vi "Write configuration.vi"(8 "error in":errorcluster, 10 "configuration":refnum<class "NISE_CEF_serializable configuration.lvclass">, 11 "cfg cRIO root in":refnum<class "cfg cRIO root.lvclass">) -> (0 "error out":errorcluster, 3 "cfg cRIO root out":refnum<class "cfg cRIO root.lvclass">)   [LabVIEW 2013, in "cfg cRIO root.lvclass"]
uses:
  cfg cRIO root.lvclass
  criocfg/crio configuration.lvclass
  CEF_TreeControl/serializable configuration/NISE_CEF_serializable configuration.lvclass
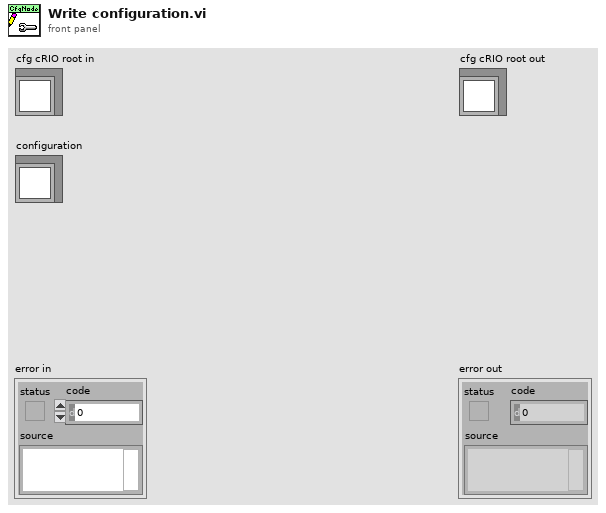
[diagram p1: front panel]
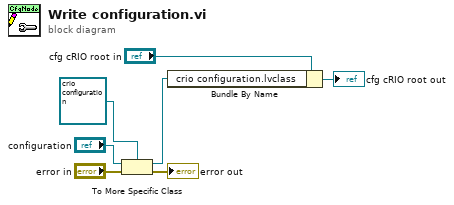
[diagram p0: block diagram]
diagram:
  n1 = To More Specific Class(target class=refnum<class "crio configuration.lvclass"> refnum ("crio configuration.lvclass"), reference="configuration", error in="error in") -> (specific class reference=w1:refnum<class "crio configuration.lvclass">, error out=→"error out":errorcluster)
  n2 = Bundle By Name(cluster="cfg cRIO root in", "crio configuration.lvclass"=w1) -> (→"cfg cRIO root out":refnum<class "cfg cRIO root.lvclass">)
